vi "test.vi"() -> ()   [LabVIEW 2019]
uses:
  <vilib>/Analysis/Matrix/Datatypes/RealMatrix.ctl
  FRC_LV_Trajectory_Library/Trajectory_Library.lvlib
  <vilib>/Analysis/Matrix/NI_Matrix.lvlib
panel:
  out "Input B":T1
  out "Input A":T1
  out "Updated B":T1
  out "B":T1
  out "A":T1
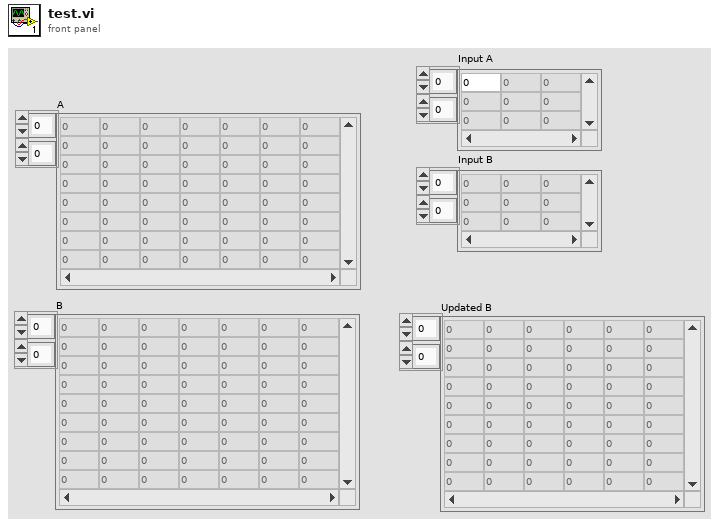
[diagram p1: front panel]
types:
  T1 = typedef "NI_Matrix.lvlib/RealMatrix.ctl" = dbl[][]
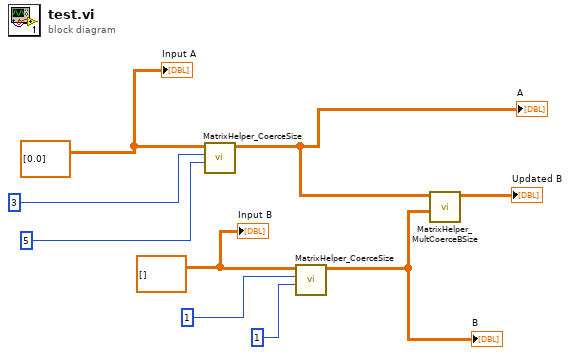
[diagram p0: block diagram]
diagram:
  w1 = T1 [] ("input matrix")
  w7 = T1 [[0.0]] ("input matrix")
  n1 = call "MatrixHelper_CoerceSize.vi"("Columns"=5, "Rows"=3, "input matrix"=w7) -> ("output matrix"=w4:T1)  [unwired: 8 in]
  "A" <- w4
  n2 = call "MatrixHelper_CoerceSize.vi"("Columns"=1, "Rows"=1, "input matrix"=w1) -> ("output matrix"=w3:T1)  [unwired: 8 in]
  "B" <- w3
  n3 = call "MatrixHelper_MultCoerceBSize.vi"("B"=w3, "A"=w4) -> ("Updated B"=→"Updated B":T1)  [unwired: 9 in]
  "Input A" <- w7
  "Input B" <- w1
